vi "Update Title.vi"(0 "Room Service Manager Model in":refnum<class "Room Service Manager Model.lvclass">, 5 "Room No":string, 11 "error in (no error)":errorcluster) -> (4 "Room Service Manager Model out":refnum<class "Room Service Manager Model.lvclass">, 15 "error out":errorcluster)   [LabVIEW 2023, in "Room Service Manager Model.lvlib" / "Room Service Manager Model.lvclass"]
uses:
  Room Service Manager Model.lvclass
  Room Service Manager Model.lvclass/Room Service Manager Model.ctl
  Room Service Manager UI/Room Service Manager UI Messages/Update Title Msg/Update Title Msg.lvclass
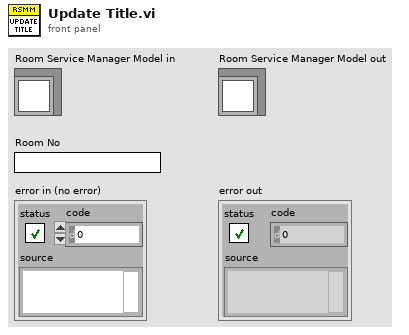
[diagram p1: front panel]
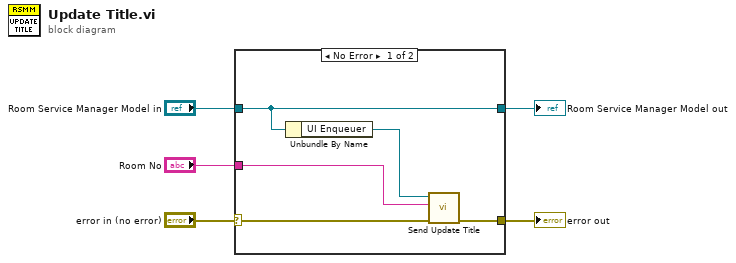
[diagram p0: block diagram]
diagram:
  n1 = case shown="No Error" "error in (no error)" {
    selector: "error in (no error)" -> [w8 w12]
    tunnel: [w7 w12] -> w2
    tunnel: [w10 w11] -> w3
    tunnel: "Room Service Manager Model in" -> [w10 w11]
    tunnel: "Room No" -> [w9 _]
    frame No Error {
      n2 = Unbundle By Name(w10) -> ("UI Enqueuer"=w6:refnum<class "Message Enqueuer.lvclass">)
      n3 = call "Send Update Title.vi"("error in (no error)"=w8, "Room No"=w9, "Message Enqueuer"=w6) -> ("error out"=w7:errorcluster)  [unwired: 7 in, 1 out]
    }
    frame Error {
    }
  }
  "error out" <- w2
  "Room Service Manager Model out" <- w3
